vi "Get Started.vi"(11 "Game in":refnum<class "Game.lvclass">) -> (2 "Started":timestamp)   [LabVIEW 2022 SP3, in "Conditum-Example.lvlib" / "Game.lvclass"]
uses:
  Game.lvclass
  Game.lvclass/Game.ctl
  Conditum/Columns/Timestamp/Timestamp.lvclass
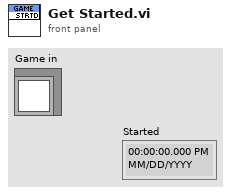
[diagram p1: front panel]
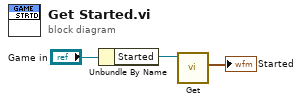
[diagram p0: block diagram]
diagram:
  n1 = Unbundle By Name("Game in") -> ("Started"=w2:refnum<class "Timestamp.lvclass">)
  n2 = call "Get.vi"("Timestamp in"=w2) -> ("Value"=→"Started":timestamp)  [unwired: 10 in]
